vi "getInfo.vi"(0 "array":dbl[](array[numeric]), 1 "srcID":u16=6, 2 "srcIDPck":u8=6) -> (3 "reliability":dbl, 4 "delay":dbl, 5 "errors":dbl, 6 "interSampling":dbl)   [LabVIEW 2009]
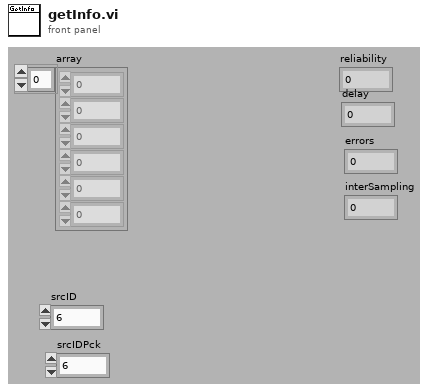
[diagram p1: front panel]
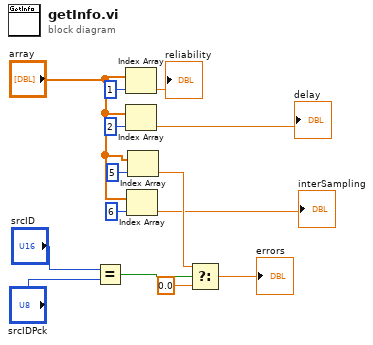
[diagram p0: block diagram]
diagram:
  n1 = Equal?(x="srcID", y="srcIDPck") -> (x = y?=w10:bool)
  n2 = Index Array(array="array", index=1) -> (element=→"reliability":dbl)
  n3 = Index Array(array="array", index=2) -> (element=→"delay":dbl)
  n4 = Index Array(array="array", index=6) -> (element=→"interSampling":dbl)
  n5 = Index Array(array="array", index=5) -> (element=w7:dbl)
  n6 = Select(t=w7, s=w10, f=0.0) -> (s? t:f=→"errors":dbl)
